vi "niDTS WLAN DSSS Tx Test UTIL DSSS Additional Limits.vi"(8 "error in (no error)":errorcluster, 9 "LSL In":T1 {"OBW"."Stop Frequency (Hz)" format="%#_4p"; "OBW"."Start Frequency (Hz)" format="%#_4p"; "OBW"."OBW (Hz)" format="%#_4p"}, 10 "USL In":T1 {"OBW"."Stop Frequency (Hz)" format="%#_4p"; "OBW"."Start Frequency (Hz)" format="%#_4p"; "OBW"."OBW (Hz)" format="%#_4p"}, 11 "Dummy Test Handle in":T16) -> (0 "error out":errorcluster, 1 "LSL":T1 {"OBW"."Stop Frequency (Hz)" format="%#_4p"; "OBW"."Start Frequency (Hz)" format="%#_4p"; "OBW"."OBW (Hz)" format="%#_4p"}, 2 "USL":T1 {"OBW"."Stop Frequency (Hz)" format="%#_4p"; "OBW"."Start Frequency (Hz)" format="%#_4p"; "OBW"."OBW (Hz)" format="%#_4p"}, 3 "Dummy Test Handle out":T16)   [LabVIEW 2015, in "niDTS WLAN.lvlib"]
uses:
  niDTS WLAN.lvlib
  Tx Test/Includes/niDTS WLAN Tx Test INC Handle.ctl
  Tx Test/Objects/BASE_class/niDTS WLAN Tx Test.lvclass
  Tx Test/Includes/niDTS WLAN Tx Test INC DSSS Results.ctl
  Tx Test/Includes/niDTS WLAN Tx Test INC DSSS MOD EVM Results.ctl
  Includes/Results/niDTS WLAN DSSS Tx RES EVM ALL.ctl
  Includes/Results/niDTS WLAN DSSS Tx RES EVM RMS.ctl
  Tx Test/Includes/niDTS WLAN Tx Test INC TXP Results.ctl
  Tx Test/Includes/niDTS WLAN Tx Test INC TXP Result SINGLE.ctl
  Tx Test/Includes/niDTS WLAN Tx Test INC OBW Results.ctl
  Instrument/INSTR TX/Results/niDTS WLAN INSTR TX INC SEM Results.ctl
  Instrument/INSTR TX/Results/niDTS WLAN INSTR TX INC SEM FSEGemts Results.ctl
  Tx Test/Includes/Results/niDTS Tx RES INC SEM FSEGemts.ctl
  Instrument/INSTR TX/Results/niDTS WLAN INSTR TX INC SEM MARGin Results.ctl
  Tx Test/Includes/Results/niDTS Tx RES INC SEM Margin.ctl
  Tx Test/Includes/niDTS WLAN Tx Test INC DSSS MOD Impairments Results.ctl
  Includes/Results/niDTS WLAN DSSS Tx Impairmentsctl.ctl
  Includes/Results/niDTS WLAN DSSS Tx PowerRamp.ctl
  Instrument/INSTR TX/niDTS WLAN INSTR TX.lvclass
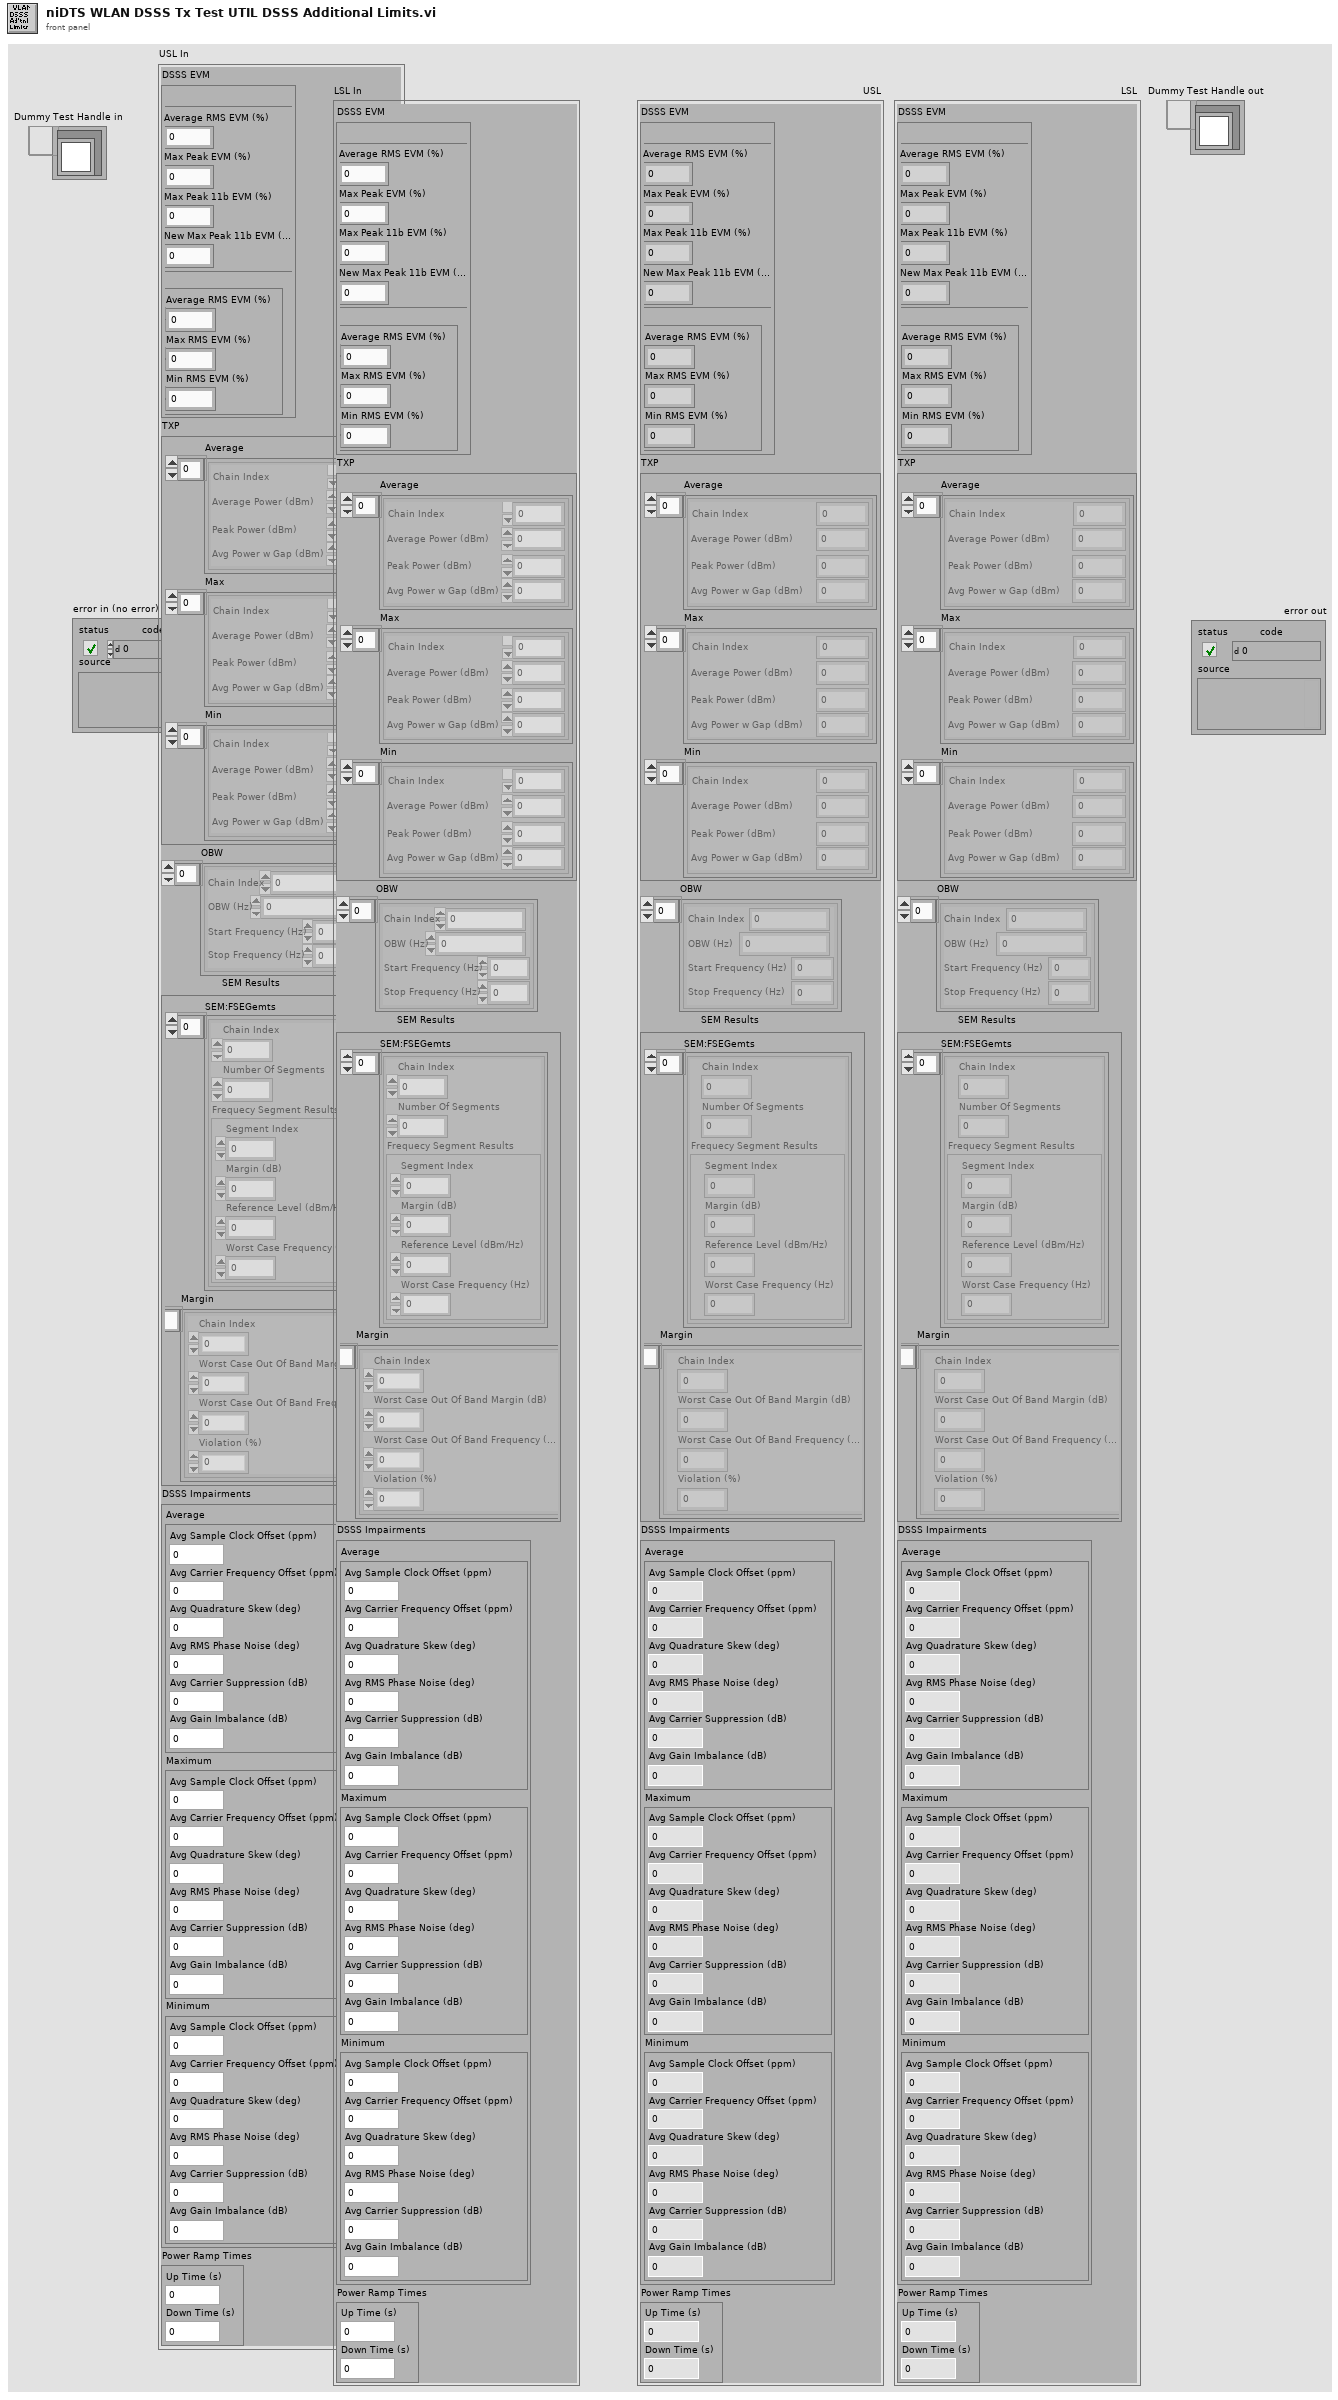
[diagram p1: front panel]
types:
  T1 = typedef "niDTS WLAN.lvlib/niDTS WLAN Tx Test INC DSSS Results.ctl" = cluster{"DSSS EVM":T2, "TXP":T5, "OBW":T7[], "SEM Results":T8, "DSSS Impairments":T13, "Power Ramp Times":T15}
  T2 = typedef "niDTS WLAN.lvlib/niDTS WLAN Tx Test INC DSSS MOD EVM Results.ctl" = cluster{"All":T3, "RMS":T4}
  T3 = typedef "niDTS WLAN.lvlib/niDTS WLAN DSSS Tx RES EVM ALL.ctl" = cluster{"Average RMS EVM (%)":dbl, "Max Peak EVM (%)":dbl, "Max Peak 11b EVM (%)":dbl, "New Max Peak 11b EVM (%)":dbl}
  T4 = typedef "niDTS WLAN.lvlib/niDTS WLAN DSSS Tx RES EVM RMS.ctl" = cluster{"Average RMS EVM (%)":dbl, "Max RMS EVM (%)":dbl, "Min RMS EVM (%)":dbl}
  T5 = typedef "niDTS WLAN.lvlib/niDTS WLAN Tx Test INC TXP Results.ctl" = cluster{"Average":T6[], "Max":T6[], "Min":T6[]}
  T6 = typedef "niDTS WLAN.lvlib/niDTS WLAN Tx Test INC TXP Result SINGLE.ctl" = cluster{"Chain Index":dbl, "Average Power (dBm)":dbl, "Peak Power (dBm)":dbl, "Avg Power w Gap (dBm)":dbl}
  T7 = typedef "niDTS WLAN.lvlib/niDTS WLAN Tx Test INC OBW Results.ctl" = cluster{"Chain Index":dbl, "OBW (Hz)":dbl, "Start Frequency (Hz)":dbl, "Stop Frequency (Hz)":dbl}
  T8 = typedef "niDTS WLAN.lvlib/niDTS WLAN INSTR TX.lvclass/niDTS WLAN INSTR TX INC SEM Results.ctl" = cluster{"SEM:FSEGemts":T9, "Margin":T11}
  T9 = typedef "niDTS WLAN.lvlib/niDTS WLAN INSTR TX.lvclass/niDTS WLAN INSTR TX INC SEM FSEGemts Results.ctl" = T10[]
  T10 = typedef "niDTS WLAN.lvlib/niDTS Tx RES INC SEM FSEGemts.ctl" = cluster{"Chain Index":i32, "Number Of Segments":i32, "Frequecy Segment Results":cluster{"Segment Index":i32, "Margin (dB)":dbl, "Reference Level (dBm/Hz)":dbl, "Worst Case Frequency (Hz)":dbl}}
  T11 = typedef "niDTS WLAN.lvlib/niDTS WLAN INSTR TX.lvclass/niDTS WLAN INSTR TX INC SEM MARGin Results.ctl" = T12[]
  T12 = typedef "niDTS WLAN.lvlib/niDTS Tx RES INC SEM Margin.ctl" = cluster{"Chain Index":i32, "Worst Case Out Of Band Margin (dB)":dbl, "Worst Case Out Of Band Frequency (Hz)":dbl, "Violation (%)":dbl}
  T13 = typedef "niDTS WLAN.lvlib/niDTS WLAN Tx Test INC DSSS MOD Impairments Results.ctl" = cluster{"Average":T14, "Maximum":T14, "Minimum":T14}
  T14 = typedef "niDTS WLAN.lvlib/niDTS WLAN DSSS Tx Impairmentsctl.ctl" = cluster{"Avg Sample Clock Offset (ppm)":dbl, "Avg Carrier Frequency Offset (ppm)":dbl, "Avg Quadrature Skew (deg)":dbl, "Avg RMS Phase Noise (deg)":dbl, "Avg Carrier Suppression (dB)":dbl, "Avg Gain Imbalance (dB)":dbl}
  T15 = typedef "niDTS WLAN.lvlib/niDTS WLAN DSSS Tx PowerRamp.ctl" = cluster{"Up Time (s)":dbl, "Down Time (s)":dbl}
  T16 = typedef "niDTS WLAN.lvlib/niDTS WLAN Tx Test INC Handle.ctl" = refnum<data-value>
  T17 = typedef "niDTS WLAN.lvlib/niDTS WLAN Tx Test INC Parameters.ctl" = cluster{"Standard":T18, "DSSS Data Rate (Mbps)":T19, "OFDM Data Rate (Mbps)":T20, "MCS Index":i32, "N spatial streams":i32, "Chains":bool[], "BandWidth (Hz)":T21, "Channel":i32, "Gard Interval":T22, "FEC Coding":T23, "Dut Tx Power":dbl, "16 symbols":bool, "payload length bytes":i32, "idle interval":dbl, "External Attenuation":dbl[], "Acquisition Parameters ":T24, "TXP Measurement Parameters":T25, "ModAcc Measurement Paramaters":T26, "ModAcc DSSS Paramaters":T27, "SEM Measurement Parameters":T29, "OBW Measurement Parameters":T30, "DSSS Power Ramp":T31, "Enable Traces":bool}
  T18 = typedef "niDTS WLAN.lvlib/niDTS WLAN INC Standard.ctl" = enum16{"802.11 b DSSS", "802.11 a/g OFDM", "802.11 n HT", "802.11 ac VHT"}
  T19 = typedef "niDTS WLAN.lvlib/niDTS WLAN INC DSSS Data Rate.ctl" = enum16{"1", "2", "5.5", "11"}
  T20 = typedef "niDTS WLAN.lvlib/niDTS WLAN INC OFDM Data Rate.ctl" = enum16{"6", "9", "12", "18", "24", "36", "48", "54"}
  T21 = typedef "niDTS WLAN.lvlib/niDTS WLAN INC CH BW.ctl" = enum16{"20 MHz", "40 MHz", "80 MHz", "160 MHz"}
  T22 = typedef "niDTS WLAN.lvlib/niDTS WLAN INC GI.ctl" = enum16{"LONG", "SHORT"}
  T23 = typedef "niDTS WLAN.lvlib/niDTS WLAN INC FEC Coding.ctl" = enum16{"BCC", "LDPC"}
  T24 = typedef "niDTS WLAN.lvlib/niDTS WLAN DUT INC Acquisition Parameters.ctl" = cluster{"Acquisition Length Mode":enum16{"AUTO", "MANUAL"}, "Acquisition Length (s)":dbl, "Auto Level":bool}
  T25 = typedef "niDTS WLAN.lvlib/niDTS WLAN INC TXP Measurement Parameters.ctl" = cluster{"TXP Power Enable":bool, "TXP Averages":i32}
  T26 = typedef "niDTS WLAN.lvlib/niDTS WLAN INC ModAcc Measurement Parameters.ctl" = cluster{"ModAcc Enable":bool, "Header Detection":enum16{"MANUAL", "FIRST", "ALL"}, "Averages":i32, "Amplitude Tracking":bool, "Channel Tracking":bool, "Time Tracking":bool, "Phase Tracking":enum16{"NONE", "STANDARD", "CSF", "INSTANT"}, "Clock Offset Est":bool, "Impairments Est":bool, "CFO Estimation":enum16{"PAMBLE", "PDATA"}}
  T27 = typedef "niDTS WLAN.lvlib/niDTS WLAN INC DSSS ModAcc Measurement Parameters.ctl" = cluster{"DC Offset Compensation":bool, "Equalization":bool, "Phase Tracking":bool, "Chip Start Location":i16, "Max Chips Used":i16, "Pulse Shaping FilterType":T28, "Pulse Shaping Filter Coefficient":dbl}
  T28 = typedef "niDTS WLAN.lvlib/niDTS WLAN INC Pulse Shaping Filter Type.ctl" = enum16{"NONE", "RCOSINE", "RRCOSINE", "GAUSSIAN"}
  T29 = typedef "niDTS WLAN.lvlib/niDTS WLAN INC SEM Measurement Parameters.ctl" = cluster{"SEM Enable":bool, "SEM Averages":i32, "Auto Span Enable":bool, "Frequency Span (Hz)":dbl, "Measurement Type":enum16{"Standard", "Legacy", "Custom"}, "Mask Frequencies (Hz)":dbl[], "Mask Power Offsets (dB)":dbl[]}
  T30 = typedef "niDTS WLAN.lvlib/niDTS WLAN INC OBW Measurement Parameters.ctl" = cluster{"OBW Enable":bool, "OBW Averages":i32}
  T31 = typedef "niDTS WLAN.lvlib/niDTS WLAN INC DSSS Power Ramp Parameters.ctl" = cluster{"Power Ramp Enable":bool, "Averages":i32, "Thresholds":cluster{"Up Low (%)":dbl, "Down Low (%)":dbl, "Up High (%)":dbl, "Down High (%)":dbl}}
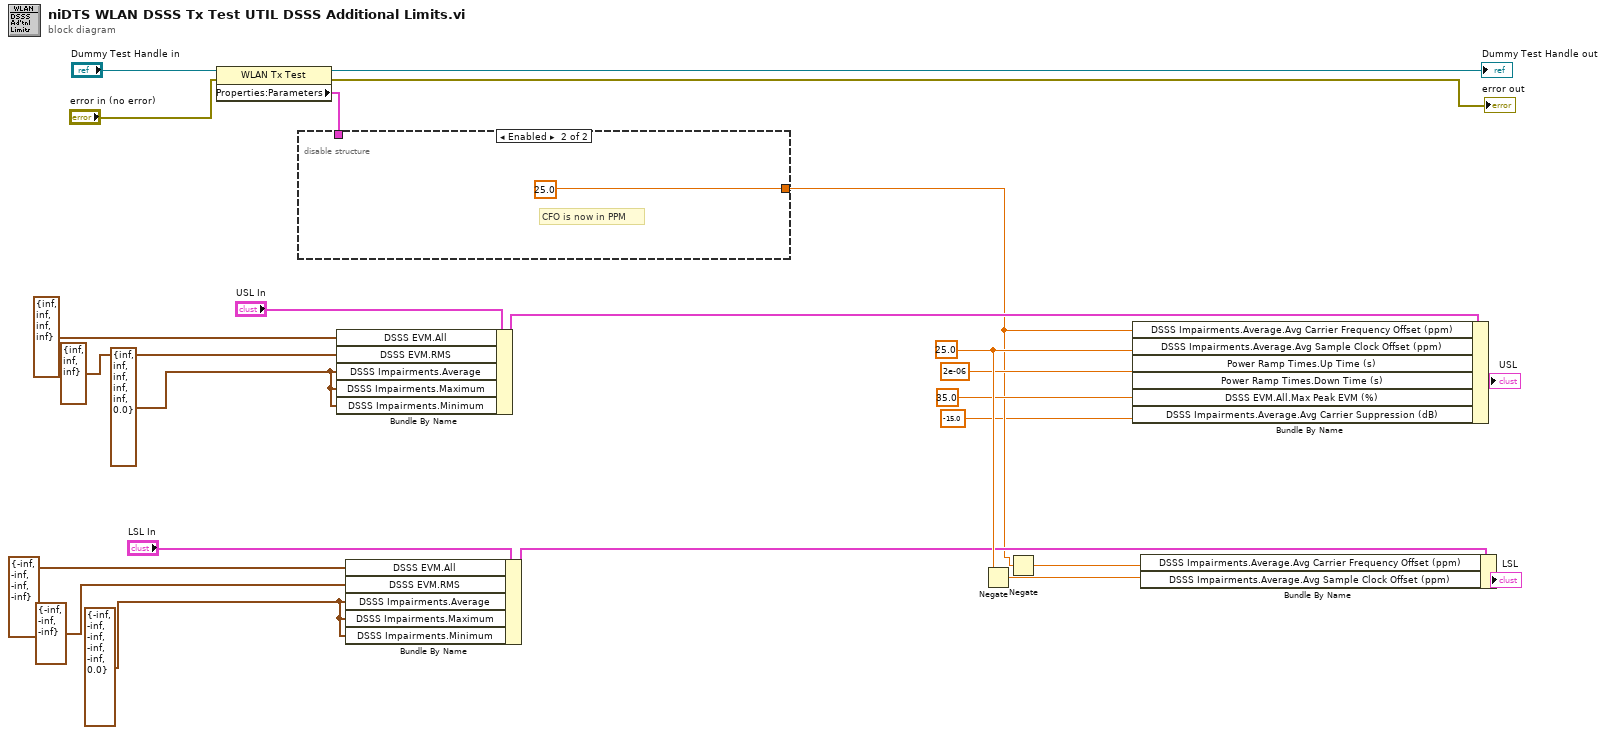
[diagram p0: block diagram]
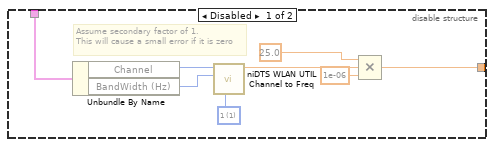
[diagram p2: hidden frame]
diagram:
  w10 = T14 {"Avg Sample Clock Offset (ppm)"=-inf, "Avg Carrier Frequency Offset (ppm)"=-inf, "Avg Quadrature Skew (deg)"=-inf, "Avg RMS Phase Noise (deg)"=-inf, "Avg Carrier Suppression (dB)"=-inf, "Avg Gain Imbalance (dB)"=0.0} ("DSSS Impairments.Average")
  w15 = T14 {"Avg Sample Clock Offset (ppm)"=inf, "Avg Carrier Frequency Offset (ppm)"=inf, "Avg Quadrature Skew (deg)"=inf, "Avg RMS Phase Noise (deg)"=inf, "Avg Carrier Suppression (dB)"=inf, "Avg Gain Imbalance (dB)"=0.0} ("DSSS Impairments.Average")
  w20 = 2e-06 ("Power Ramp Times.UpTime")
  w23 = 25.0 ("DSSS Impairments.Average.AvgSampleClockOffset")
  n1 = property class="WLAN Tx Test"(reference="Dummy Test Handle in", error in="error in (no error)") -> (reference out=→"Dummy Test Handle out":T16, error out=→"error out":errorcluster, "Properties:Parameters"=w21:T17)
  n2 = disable-structure shown="Enabled" {
    disable-tunnel: w21 -> [w27 _]
    disable-tunnel: [w25 25.0 ("DSSS Impairments.Average.AvgSampleClockOffset")] -> w3
    frame Disabled {
      w30 = 1 items=["-1"=-1, "1"=1, "0"=0] ("secondary factor")
      # "Assume secondary factor of 1.\nThis will cause a small error if it is zero"
      n3 = Unbundle By Name(w27) -> ("Channel"=w32:i32, "BandWidth (Hz)"=w31:T21)
      n4 = call "niDTS WLAN UTIL Channel to Freq.vi"("secondary factor"=w30, "CH BW"=w31, "Channel"=w32) -> ("Center Frequency (Hz)"=w29:dbl)  [unwired: 6 in, 2 out]
      n5 = Compound Arithmetic op=MULTIPLY(25.0 ("DSSS Impairments.Average.AvgSampleClockOffset"), w29, 1e-06 ("value")) -> (w25:dbl)
    }
    frame Enabled {
      # "CFO is now in PPM"
    }
  }
  n6 = Bundle By Name(cluster="USL In", "DSSS EVM.All"=T3 {"Average RMS EVM (%)"=inf, "Max Peak EVM (%)"=inf, "Max Peak 11b EVM (%)"=inf, "New Max Peak 11b EVM (%)"=inf}, "DSSS EVM.RMS"=T4 {"Average RMS EVM (%)"=inf, "Max RMS EVM (%)"=inf, "Min RMS EVM (%)"=inf}, "DSSS Impairments.Average"=w15, "DSSS Impairments.Maximum"=w15, "DSSS Impairments.Minimum"=w15) -> (w17:T1)
  n7 = Bundle By Name(cluster="LSL In", "DSSS EVM.All"=T3 {"Average RMS EVM (%)"=-inf, "Max Peak EVM (%)"=-inf, "Max Peak 11b EVM (%)"=-inf, "New Max Peak 11b EVM (%)"=-inf}, "DSSS EVM.RMS"=T4 {"Average RMS EVM (%)"=-inf, "Max RMS EVM (%)"=-inf, "Min RMS EVM (%)"=-inf}, "DSSS Impairments.Average"=w10, "DSSS Impairments.Maximum"=w10, "DSSS Impairments.Minimum"=w10) -> (w13:T1)
  n8 = Negate(x=w23) -> (-x=w24:dbl)
  n9 = Negate(x=w3) -> (-x=w2:dbl)
  n10 = Bundle By Name(cluster=w17, "DSSS Impairments.Average.Avg Carrier Frequency Offset (ppm)"=w3, "DSSS Impairments.Average.Avg Sample Clock Offset (ppm)"=w23, "Power Ramp Times.Up Time (s)"=w20, "Power Ramp Times.Down Time (s)"=w20, "DSSS EVM.All.Max Peak EVM (%)"=35.0 ("DSSS EVM.All.MaxPeakEvm"), "DSSS Impairments.Average.Avg Carrier Suppression (dB)"=-15.0 ("DSSS Impairments.Average.AvgCarrierSuppression")) -> (→"USL":T1)
  n11 = Bundle By Name(cluster=w13, "DSSS Impairments.Average.Avg Carrier Frequency Offset (ppm)"=w2, "DSSS Impairments.Average.Avg Sample Clock Offset (ppm)"=w24) -> (→"LSL":T1)
